vi "FractalNet BaseStation with GPS Weather and Gesture Display.vi"() -> ()   [LabVIEW 2009]
doc: "This example demonstrates some fundamental concepts for the 3D picture control. Concepts covered include:\n\n-Object creation\n-Texturing\n-Object movement\n-Object hierarchy"
uses:
  <vilib>/Utility/miscctls.llb/LVRectTypeDef.ctl
  <vilib>/Instr/_visa.llb/VISA Configure Serial Port (Instr).vi
  <vilib>/regexp/Match Regular Expression.xnode
  <vilib>/Analysis/coordinate.llb/3D Cartesian Coordinate Rotation (Euler) (Array).vi
  <vilib>/picture/3D Picture Control/NI_3D Picture Control.lvlib
  <vilib>/Analysis/NI_AALPro.lvlib
  <vilib>/Platform/NI_3dgraph.lvlib
panel:
  in  "3D Surface":refnum<k7>(container)
  out "Thermometer":dbl(slide) scale=0.0..100.0
  out "Status":dbl(knob)=5.599555604389847 scale=0.0..10.0
  in  "Boolean 7":bool
  out "Boolean 6":bool
  out "Boolean 5":bool
  out "Boolean 4":bool
  in  "Boolean 3":bool=TRUE
  in  "Boolean 2":bool=TRUE
  in  "Boolean":bool
  in  "Control":dbl(knob)=2.859770666370601 scale=0.0..10.0
  out "DENIO - CAVE 1":dbl(knob) scale=600.0..480.0
  out "GREENE - CAVE 2":dbl(knob) scale=600.0..480.0
  out "VAUGHN - SHIP":dbl(knob) scale=600.0..480.0
  in  "Acquire Glove":bool
  out "Date":string
  out "Base Heading (degrees)":dbl
  out "Base speed (mph)":dbl
  out "Time":string
  out "Longitude":string
  out "Latitude":string
  out "# of satellites":string
  out "Altitude (ft)":string
  out "Outside Pressure":string
  out "Outside Temp (F)":string
  out "Outside Temp (C)":string
  out "Outside Humidity":string
  in  "COMM for GPS / Weather":refnum<visa-resource-name>="COM22"
  in  "VISA Resource Name":refnum<visa-resource-name>="COM24"
  out "Raw DataGlove String":string
  out "Yaw":string
  out "Pitch":string
  out "Roll":string
  out "Heart":string
  out "Thumb":dbl(slide) scale=780.0..815.0
  out "Index":dbl(slide) scale=518.0..735.0
  out "Middle":dbl(slide) scale=780.0..880.0
  out "Ring":dbl(slide) scale=720.0..870.0
  in  "Render Dest":enum16{"Scene Window", "Scene Display"}(ring)=enum."Scene Display"
  in  "Camera Controller":enum16{"None", "Spherical", "Flying"}(ring)=enum."Spherical"
  out "Scene Display":refnum<vi>(3d-picture)
  out "error out":errorcluster
  in  "stop":bool
  # "NODE MAP STATUS"
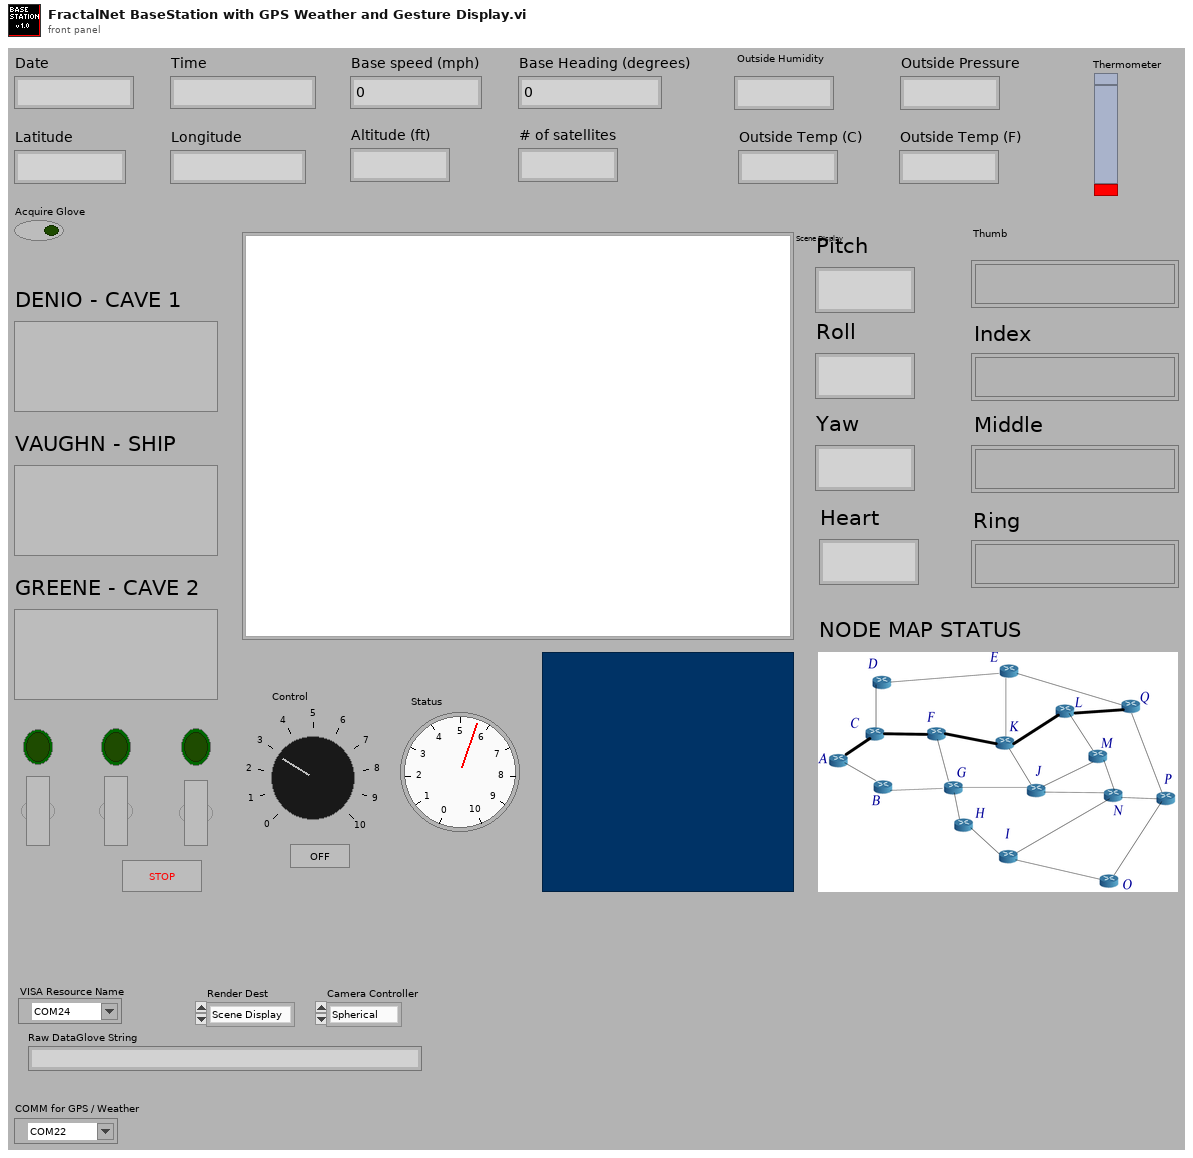
[diagram p1: front panel]
types:
  T1 = typedef "LVRectTypeDef.ctl" = cluster{"Left":i16, "Top":i16, "Right":i16, "Bottom":i16}
  T2 = enum16{"Open", "Minimized", "Maximized", "Hidden"}
  T3 = enum16{"As a Decal", "With Modulation", "With Blending", "As a replacement"}
  T4 = typedef "imagedata.ctl" = cluster{"image type":i32, "image depth":i32, "image":u8[], "mask":u8[], "colors":u32[], "Rectangle":cluster{"left":i16, "top":i16, "right":i16, "bottom":i16}}
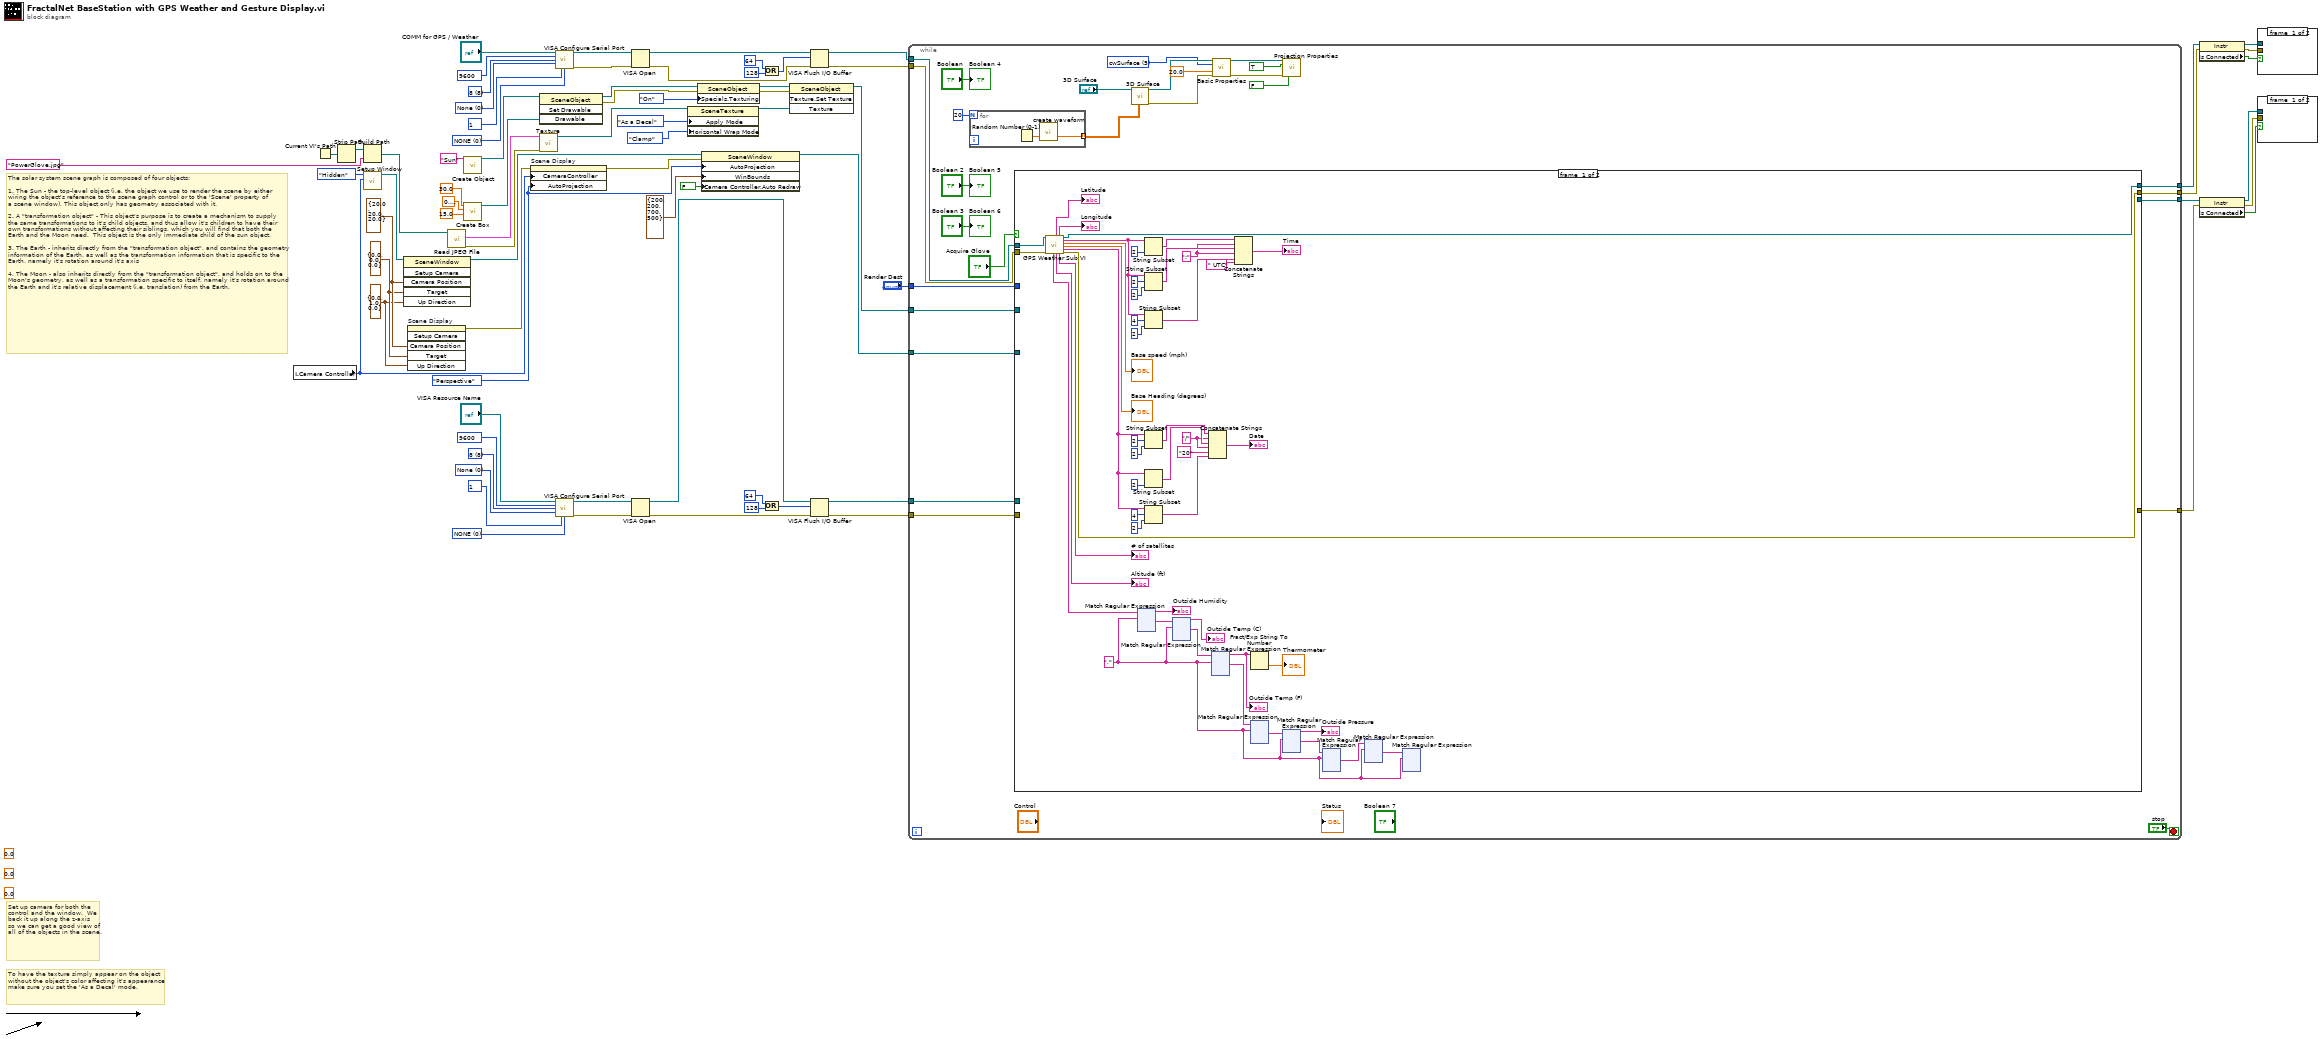
[diagram p0: block diagram]
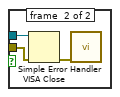
[diagram p2: hidden frame]
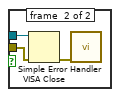
[diagram p3: hidden frame]
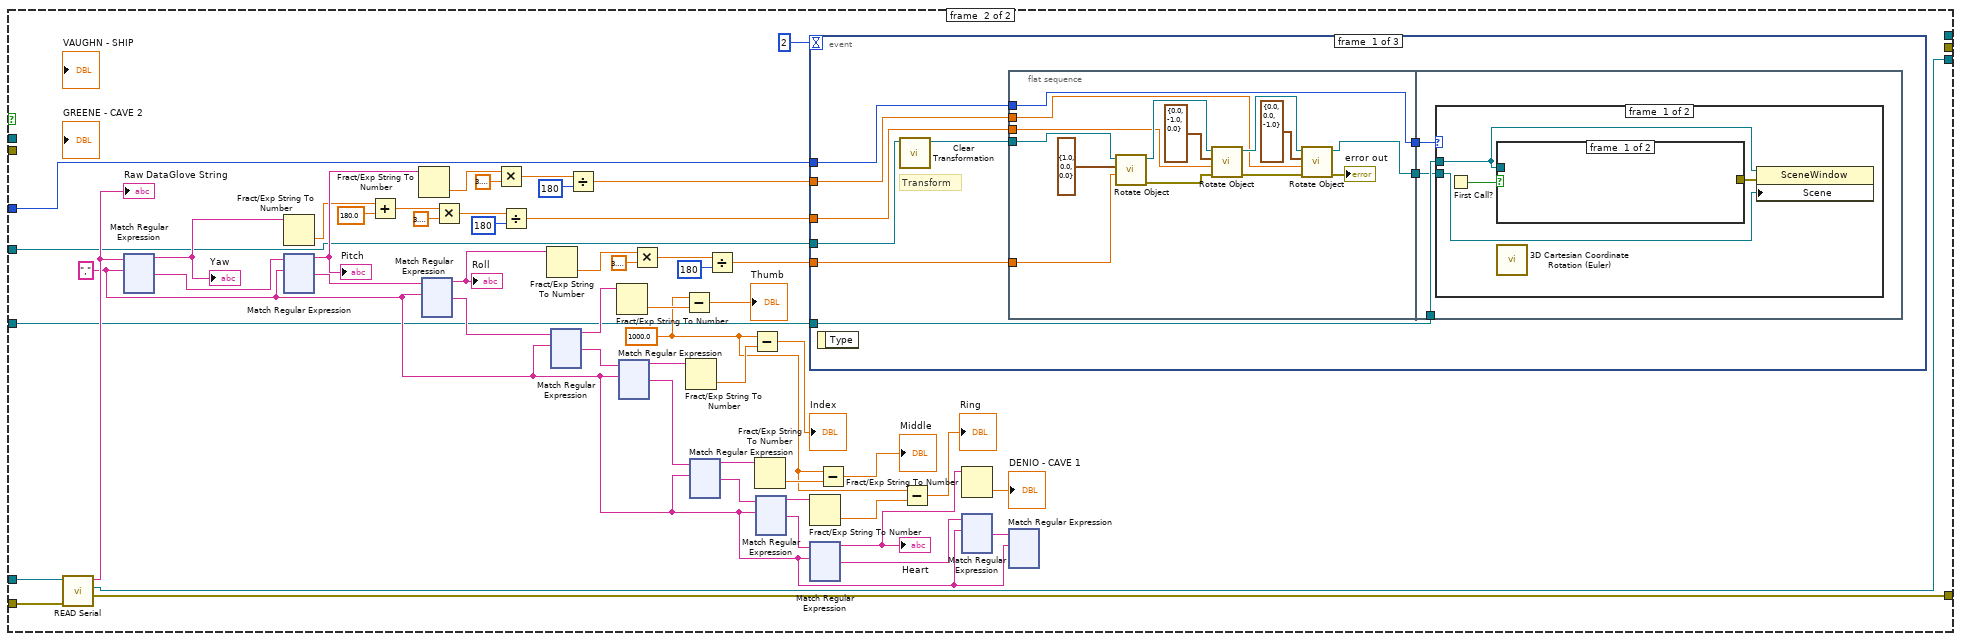
[diagram p4: hidden frame]
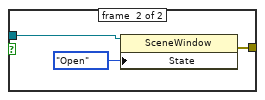
[diagram p5: hidden frame]
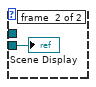
[diagram p6: hidden frame]
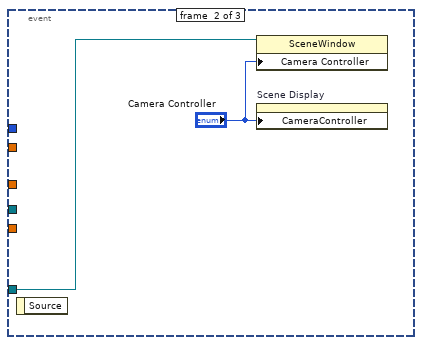
[diagram p7: hidden frame]
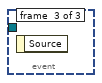
[diagram p8: hidden frame]
diagram:
  w13 = u16 0 items=["NONE", "XON/XOFF", "RTS/CTS", "XON/XOFF & RTS/CTS", "DTR/DSR", "XON/XOFF & DTR/DSR"] ("flow control")
  w14 = u16 10 items=["1"=10, "1.5"=15, "2"=20] ("stop bits")
  w15 = u16 0 items=["None", "Odd", "Even", "Mark", "Space"] ("parity")
  w16 = u16 8 items=["8"=8, "7"=7, "6"=6, "5"=5] ("data bits")
  w17 = u32 9600 items=["1200"=1200, "2400"=2400, "4800"=4800, "9600"=9600, "19200"=19200, "38400"=38400, "57600"=57600, "115200"=115200] ("baud rate")
  (unwired) 0.0
  (unwired) 0.0
  (unwired) 0.0
  w34 = u16 0 items=["NONE", "XON/XOFF", "RTS/CTS", "XON/XOFF & RTS/CTS", "DTR/DSR", "XON/XOFF & DTR/DSR"] ("flow control")
  w35 = u16 10 items=["1"=10, "1.5"=15, "2"=20] ("stop bits")
  w36 = u16 0 items=["None", "Odd", "Even", "Mark", "Space"] ("parity")
  w37 = u16 8 items=["8"=8, "7"=7, "6"=6, "5"=5] ("data bits")
  w38 = u32 9600 items=["1200"=1200, "2400"=2400, "4800"=4800, "9600"=9600, "19200"=19200, "38400"=38400, "57600"=57600, "115200"=115200] ("baud rate")
  w53 = enum16{"None", "Perspective", "Orthographic"}."Perspective" ("Auto Projection Mode")
  w56 = cluster{"X":sgl, "Y":sgl, "Z":sgl} {"X"=0.0, "Y"=1.0, "Z"=0.0} ("Up Direction")
  w57 = cluster{"X":sgl, "Y":sgl, "Z":sgl} {"X"=0.0, "Y"=0.0, "Z"=0.0} ("Target")
  w58 = cluster{"X":sgl, "Y":sgl, "Z":sgl} {"X"=20.0, "Y"=20.0, "Z"=20.0} ("Camera Position")
  # "Set up camera for both the \ncontrol and the window.  We\nback it up along the z-axis\nso we can get a good view of\nall of the objects in the scene."
  # "To have the texture simply appear on the object\nwithout the object's color affecting it's appearance\nmake sure you set the 'As a Decal' mode."
  # "The solar system scene graph is composed of four objects:\n\n1. The Sun - the top-level object (i.e. the object we use to render the scene by either\nwiring the object's reference to the scene graph control or to the 'Scene' property of \na scene window). This object only has geometry associated with it.\n\n2. A \"transformation object\" - This object's purpose is to create a mechanism to supply\nthe same transformations to it's child objects, and thus allow it's children to have their\nown transformations without affecting their siblings, which you will find that both the \nEarth and the Moon need.  This object is the only immediate child of the sun object.\n\n3. The Earth - inherits directly from the \"transformation object\", and contains the geometry\ninformation of the Earth, as well as the transformation information that is specific to the \nEarth, namely it's rotation around it's axis\n\n4. The Moon - also inherits directly from the \"transformation object\", and holds on to the \nMoon's geometry, as well as a transformation specific to itself, namely it's rotation around\nthe Earth and it's relative displacement (i.e. translation) from the Earth."
  n1 = local read "Camera Controller"() -> (w49:enum16{"None", "Spherical", "Flying"})
  n2 = Current VI's Path() -> (path=w63:path)
  n3 = Strip Path(path=w63) -> (stripped path=w62:path)  [unwired: 1 out]
  n4 = Build Path(base path=w62, name or relative path="PowerGlove.jpg" ("Name")) -> (appended path=w60:path)
  n5 = call <vilib>:"Setup Window.vi"("Camera Controller"=w49, "Window State"=T2."Hidden") -> ("New Window Refnum"=w51:refnum<vi>)  [unwired: 1 in, 8 out]
  n6 = invoke class="SceneWindow" method="Setup Camera"(reference=w51, "Camera Position"=w58, "Target"=w57, "Up Direction"=w56) -> (reference out=w76:refnum<vi>)  [unwired: 2 in, 5 out]
  n7 = invoke on="Scene Display" class="SceneGraphDisp (strict)" method="Setup Camera"("Camera Position"=w58, "Target"=w57, "Up Direction"=w56) -> (error out=w55:errorcluster)  [unwired: 3 in, 5 out]
  n8 = call <vilib>:"Read JPEG File.vi"("path to JPEG file"=w60) -> ("error out"=w72:errorcluster, "image data"=w73:T4)  [unwired: 1 in, 8 out]
  n9 = call <vilib>:"Create Object.vi"("Name"="Sun") -> ("Scene:New Object"=w74:refnum<vi>)  [unwired: 1 in, 9 out]
  n10 = call <vilib>:"Create Box.vi"("Length Z"=sgl 15.0, "Length Y"=sgl 0.1, "Length X"=sgl 30.0) -> ("New Box Refnum"=w42:refnum<vi>)  [unwired: 7 in, 1 out]
  n11 = property on="Scene Display" class="SceneGraphDisp (strict)"(error in=w55, "CameraController"=w49, "AutoProjection"=w53) -> (error out=w54:errorcluster)  [unwired: 1 in, 1 out]
  n12 = call <vilib>:"Texture.vi"("error in (no error)"=w72, "Image"=w73) -> ("New Texture Refnum"=w66:refnum<vi>)  [unwired: 9 out]
  n13 = invoke class="SceneObject" method="Set Drawable"(reference=w74, "Drawable"=w42) -> (reference out=w71:refnum<vi>, error out=w69:errorcluster)  [unwired: 2 in, 2 out]
  n14 = call-poly "VISA Configure Serial Port"("VISA resource name"="COMM for GPS / Weather", "baud rate (9600)"=w17, "data bits (8)"=w16, "parity (0:none)"=w15, "stop bits (10: 1 bit)"=w14, "flow control (0:none)"=w13) -> ("VISA resource name out"=w20:refnum<visa-resource-name>, "error out"=w19:errorcluster)  [unwired: 1 in, 7 out]
  n15 = call-poly "VISA Configure Serial Port"("VISA resource name"="VISA Resource Name", "baud rate (9600)"=w38, "data bits (8)"=w37, "parity (0:none)"=w36, "stop bits (10: 1 bit)"=w35, "flow control (0:none)"=w34) -> ("VISA resource name out"=w41:refnum<visa-resource-name>, "error out"=w40:errorcluster)  [unwired: 1 in, 7 out]
  n16 = VISA Open(error in (no error)=w19, VISA resource name=w20) -> (VISA resource name=w12:refnum<visa-resource-name>, error out=w11:errorcluster)  [unwired: 3 out]
  n17 = VISA Open(error in (no error)=w40, VISA resource name=w41) -> (VISA resource name=w33:refnum<visa-resource-name>, error out=w32:errorcluster)  [unwired: 3 out]
  n18 = property class="SceneTexture"(reference=w66, "Apply Mode"=T3."As a Decal", "Horizontal Wrap Mode"=enum16{"Clamp", "Repeat"}."Clamp") -> (reference out=w64:refnum<vi>)  [unwired: 1 in, 1 out]
  n19 = property class="SceneObject"(reference=w71, error in=w69, "Specials.Texturing"=enum16{"Inherit Value", "Off", "On"}."On" ("Specials:Texturing")) -> (reference out=w70:refnum<vi>, error out=w68:errorcluster)
  n20 = property class="SceneWindow"(reference=w76, error in=w54, "AutoProjection"=w53, "WinBounds"=T1 {"Left"=200, "Top"=200, "Right"=700, "Bottom"=500} ("Window Bounds"), "Camera Controller.Auto Redraw"=FALSE ("Camera Controller:Auto Redraw")) -> (reference out=w47:refnum<vi>)  [unwired: 1 out]
  n21 = Compound Arithmetic op=OR(64, 128) -> (w8:i32)
  n22 = Compound Arithmetic op=OR(64, 128) -> (w29:i32)
  n23 = invoke class="SceneObject" method="Texture.Set Texture"(reference=w70, error in=w68, "Texture"=w64) -> (reference out=w21:refnum<vi>)  [unwired: 1 in, 3 out]
  n24 = VISA Flush I/O Buffer(VISA resource name=w12, mask (16)=w8, error in (no error)=w11) -> (VISA resource name out=w7:refnum<visa-resource-name>, error out=w6:errorcluster)
  n25 = VISA Flush I/O Buffer(VISA resource name=w33, mask (16)=w29, error in (no error)=w32) -> (VISA resource name out=w23:refnum<visa-resource-name>, error out=w22:errorcluster)
  n26 = while {
    tunnel: w47 -> [w97]
    tunnel: "Render Dest" -> [w103]
    tunnel: w21 -> [w98]
    tunnel: [w102] -> w25
    tunnel: [w101] -> w24
    tunnel: w23 -> [w100]
    tunnel: w22 -> [w99]
    tunnel: w7 -> [w95]
    tunnel: w6 -> [w94]
    tunnel: [w93] -> w2
    tunnel: [w92] -> w1
    stop <- "stop" stop-if-true
    w80 = 5 items=["cwLine"=1, "cwPoint"=2, "cwLinePoint"=3, "cwHiddenLine"=4, "cwSurface"=5, "cwSurfaceLine"=6, "cwSurfaceNormal"=7, "cwContourLine"=8, "cwSurfaceContour"=9] ("Plot Style")
    n27 = for {
      N: 20 -> [_]
      tunnel: [w104] -> w84 mode=indexing
      n28 = Random Number (0-1)() -> (number: 0 to 1=w105:dbl)
      n29 = call "create waveform.vi"("amplitude (1.0)"=w105) -> ("waveform graph"=w104:ext[])  [unwired: 13 in, 1 out]
    }
    n30 = case shown="False" "Acquire Glove" {
      tunnel: w103 -> [_ w1062]
      tunnel: [_ w1061] -> w102
      tunnel: [_ w1060] -> w101
      tunnel: w100 -> [_ w1059]
      tunnel: w99 -> [_ w1058]
      tunnel: w98 -> [_ w1013]
      tunnel: w97 -> [_ w1012]
      tunnel: w95 -> [w112 _]
      tunnel: w94 -> [w111 _]
      tunnel: [w110 _] -> w93
      tunnel: [w109 _] -> w92
      frame #0 {
        w147 = "/" ("string")
        w133 = ":" ("string")
        w138 = "," ("regular expression")
        n31 = call "GPS Weather Sub VI.vi"("VISA resource name out"=w112, "error out"=w111) -> ("Weather"=w141:string, "Latitude"=→"Latitude":string, "Altitude"=→"Altitude (ft)":string, "Longitude"=→"Longitude":string, "# of satellites"=→"# of satellites":string, "VISA resource name out 2"=w110:refnum<visa-resource-name>, "Time"=w130:string, "Base speed (mph)"=→"Base speed (mph)":dbl, "Base Heading (degrees)"=→"Base Heading (degrees)":dbl, "Date"=w148:string, "error IO"=w109:errorcluster)  [unwired: 7 in]
        n32 = xnode "Match Regular Expression"("input string"=w141, "regular expression"=w138) -> ("before match"=→"Outside Humidity":string, "after match"=w119:string)  [unwired: 2 in, 5 out]
        n33 = String Subset(string=w130, length (rest)=2 ("length (rest)")) -> (substring=w132:string)  [unwired: 1 in]
        n34 = String Subset(string=w130, offset (0)=2, length (rest)=2 ("length (rest)")) -> (substring=w134:string)
        n35 = String Subset(string=w130, offset (0)=4, length (rest)=2 ("length (rest)")) -> (substring=w135:string)
        n36 = String Subset(string=w148, offset (0)=2, length (rest)=2 ("length (rest)")) -> (substring=w149:string)
        n37 = String Subset(string=w148, length (rest)=2 ("length (rest)")) -> (substring=w150:string)  [unwired: 1 in]
        n38 = String Subset(string=w148, offset (0)=4, length (rest)=2 ("length (rest)")) -> (substring=w152:string)
        n39 = xnode "Match Regular Expression"("input string"=w119, "regular expression"=w138) -> ("before match"=→"Outside Temp (C)":string, "after match"=w118:string)  [unwired: 2 in, 5 out]
        n40 = Concatenate Strings(w149, w147, w150, w147, "20" ("string"), w152) -> (→"Date":string)
        n41 = xnode "Match Regular Expression"("input string"=w118, "regular expression"=w138) -> ("before match"=w106:string, "after match"=w117:string)  [unwired: 2 in, 5 out]
        "Outside Temp (F)" <- w106
        n42 = Concatenate Strings(w132, w133, w134, w133, w135, " UTC" ("string")) -> (→"Time":string)
        n43 = Fract/Exp String To Number(string=w106) -> (number=→"Thermometer":dbl)  [unwired: 3 in, 1 out]
        n44 = xnode "Match Regular Expression"("input string"=w117, "regular expression"=w138) -> ("after match"=w116:string)  [unwired: 2 in, 6 out]
        n45 = xnode "Match Regular Expression"("input string"=w116, "regular expression"=w138) -> ("before match"=→"Outside Pressure":string, "after match"=w115:string)  [unwired: 2 in, 5 out]
        n46 = xnode "Match Regular Expression"("input string"=w115, "regular expression"=w138) -> ("after match"=w114:string)  [unwired: 2 in, 6 out]
        n47 = xnode "Match Regular Expression"("input string"=w114, "regular expression"=w138) -> ("after match"=w113:string)  [unwired: 2 in, 6 out]
        n48 = xnode "Match Regular Expression"("input string"=w113, "regular expression"=w138) -> ()  [unwired: 2 in, 7 out]
      }
      frame #1 {
        w1036 = 1000.0 ("x")
        w1034 = "," ("regular expression")
        n49 = call "READ Serial.vi"("error in"=w1058, "VISA Resource Name In"=w1059) -> ("error out"=w1060:errorcluster, "VISA Resource Name Out"=w1061:refnum<visa-resource-name>, "Output String"=w1048:string)  [unwired: 4 in]
        "Raw DataGlove String" <- w1048
        n50 = xnode "Match Regular Expression"("input string"=w1048, "regular expression"=w1034) -> ("before match"=w1020:string, "after match"=w1057:string)  [unwired: 2 in, 5 out]
        "Yaw" <- w1020
        n51 = Fract/Exp String To Number(string=w1020) -> (number=w1016:dbl)  [unwired: 3 in, 1 out]
        n52 = xnode "Match Regular Expression"("input string"=w1057, "regular expression"=w1034) -> ("before match"=w1033:string, "after match"=w1056:string)  [unwired: 2 in, 5 out]
        "Pitch" <- w1033
        n53 = Add(x=w1016, y=180.0) -> (x+y=w1014:dbl)
        n54 = Fract/Exp String To Number(string=w1033) -> (number=w1022:dbl)  [unwired: 3 in, 1 out]
        n55 = xnode "Match Regular Expression"("input string"=w1056, "regular expression"=w1034) -> ("before match"=w1032:string, "after match"=w1055:string)  [unwired: 2 in, 5 out]
        "Roll" <- w1032
        n56 = Multiply(x=w1014, y=3.141592653589793) -> (x*y=w1030:dbl)
        n57 = Multiply(x=w1022, y=3.141592653589793) -> (x*y=w1027:dbl)
        n58 = Divide(x=w1030, y=180) -> (x/y=w1017:dbl)
        n59 = Fract/Exp String To Number(string=w1032) -> (number=w1021:dbl)  [unwired: 3 in, 1 out]
        n60 = xnode "Match Regular Expression"("input string"=w1055, "regular expression"=w1034) -> ("before match"=w1047:string, "after match"=w1050:string)  [unwired: 2 in, 5 out]
        n61 = Divide(x=w1027, y=180) -> (x/y=w1019:dbl)
        n62 = Fract/Exp String To Number(string=w1047) -> (number=w1046:dbl)  [unwired: 3 in, 1 out]
        n63 = xnode "Match Regular Expression"("input string"=w1050, "regular expression"=w1034) -> ("before match"=w1044:string, "after match"=w1054:string)  [unwired: 2 in, 5 out]
        n64 = Multiply(x=w1021, y=3.141592653589793) -> (x*y=w1024:dbl)
        n65 = Subtract(x=w1036, y=w1046) -> (x-y=→"Thumb":dbl)
        n66 = Fract/Exp String To Number(string=w1044) -> (number=w1043:dbl)  [unwired: 3 in, 1 out]
        n67 = xnode "Match Regular Expression"("input string"=w1054, "regular expression"=w1034) -> ("before match"=w1037:string, "after match"=w1053:string)  [unwired: 2 in, 5 out]
        n68 = Divide(x=w1024, y=180) -> (x/y=w1018:dbl)
        n69 = Subtract(x=w1036, y=w1043) -> (x-y=→"Index":dbl)
        n70 = Fract/Exp String To Number(string=w1037) -> (number=w1039:dbl)  [unwired: 3 in, 1 out]
        n71 = xnode "Match Regular Expression"("input string"=w1053, "regular expression"=w1034) -> ("before match"=w1040:string, "after match"=w1052:string)  [unwired: 2 in, 5 out]
        n72 = event shown="[2] \"stop\": Value Change" {
          selector: _ -> [_ _ _]
          dyn-events: _ -> [_ _ _]
          timeout: 2 -> [_ _ _]
          tunnel: w1012 -> [w2142 w2169 _]
          tunnel: w1062 -> [w2140 _ _]
          tunnel: w1013 -> [w2135 _ _]
          tunnel: w1017 -> [w2138 _ _]
          tunnel: w1018 -> [w2137 _ _]
          tunnel: w1019 -> [w2136 _ _]
          event #0 {
            # "Transform"
            n73 = event-data() -> ()  [unwired: 2 out]
            n74 = call <vilib>:"Clear Transformation.vi"("Object Refnum In"=w2135) -> ("Object Refnum Out"=w2134:refnum<vi>)  [unwired: 9 in, 1 out]
            n75 = flat-sequence {
              tunnel: w2134 -> [w2149]
              tunnel: [w2156] -> w2141
              tunnel: w2140 -> [w2156]
              tunnel: [w2150] -> w2139
              tunnel: w2138 -> [w2144]
              tunnel: w2137 -> [w2145]
              tunnel: w2136 -> [w2143]
              tunnel: w2142 -> [w2159]
              tunnel: w2141 -> [w2158]
              tunnel: w2139 -> [w2157]
              frame #0 {
                n76 = call <vilib>:"Rotate Object.vi"("Angle"=w2145, "Axis"=cluster{"X":sgl, "Y":sgl, "Z":sgl} {"X"=1.0, "Y"=0.0, "Z"=0.0}, "Scene.Object In"=w2149) -> ("error out"=w2147:errorcluster, "Scene.Object Out"=w2146:refnum<vi>)  [unwired: 7 in]
                n77 = call <vilib>:"Rotate Object.vi"("error in (no error)"=w2147, "Angle"=w2144, "Axis"=cluster{"X":sgl, "Y":sgl, "Z":sgl} {"X"=0.0, "Y"=-1.0, "Z"=0.0}, "Scene.Object In"=w2146) -> ("error out"=w2152:errorcluster, "Scene.Object Out"=w2153:refnum<vi>)  [unwired: 6 in]
                n78 = call <vilib>:"Rotate Object.vi"("error in (no error)"=w2152, "Angle"=w2143, "Axis"=cluster{"X":sgl, "Y":sgl, "Z":sgl} {"X"=0.0, "Y"=0.0, "Z"=-1.0}, "Scene.Object In"=w2153) -> ("error out"=→"error out":errorcluster, "Scene.Object Out"=w2150:refnum<vi>)  [unwired: 6 in]
              }
              frame #1 {
                n79 = case shown="\"Scene Window\", Default" w2158 {
                  tunnel: w2159 -> [w2163 _]
                  tunnel: w2157 -> [w2160 w2167]
                  frame #0 {
                    n80 = First Call?() -> (First Call?: T/F=w2161:bool)
                    n81 = case shown="True" w2161 {
                      tunnel: w2163 -> [_ w2166]
                      tunnel: [_ w2165] -> w2162
                      frame #0 {
                      }
                      frame #1 {
                        n82 = property class="SceneWindow"(reference=w2166, "State"=T2."Open" ("Window State")) -> (error out=w2165:errorcluster)  [unwired: 1 in, 1 out]
                      }
                    }
                    n83 = call-poly <vilib>:"3D Cartesian Coordinate Rotation (Euler).vi"() -> ()  [unwired: 8 in, 4 out]
                    n84 = property class="SceneWindow"(reference=w2163, error in=w2162, "Scene"=w2160) -> ()  [unwired: 2 out]
                  }
                  frame #1 {
                    "Scene Display" <- w2167
                  }
                }
              }
            }
          }
          event #1 {
            n85 = event-data() -> ()  [unwired: 2 out]
            n86 = property class="SceneWindow"(reference=w2169, "Camera Controller"="Camera Controller") -> ()  [unwired: 1 in, 2 out]
            n87 = property on="Scene Display" class="SceneGraphDisp (strict)"("CameraController"="Camera Controller") -> ()  [unwired: 2 in, 2 out]
          }
          event #2 {
            n88 = event-data() -> ()  [unwired: 2 out]
          }
        }
        n89 = Fract/Exp String To Number(string=w1040) -> (number=w1041:dbl)  [unwired: 3 in, 1 out]
        n90 = xnode "Match Regular Expression"("input string"=w1052, "regular expression"=w1034) -> ("before match"=w1011:string, "after match"=w1051:string)  [unwired: 2 in, 5 out]
        "Heart" <- w1011
        n91 = Subtract(x=w1036, y=w1039) -> (x-y=→"Middle":dbl)
        n92 = Subtract(x=w1036, y=w1041) -> (x-y=→"Ring":dbl)
        n93 = Fract/Exp String To Number(string=w1011) -> (number=→"DENIO - CAVE 1":dbl)  [unwired: 3 in, 1 out]
        n94 = xnode "Match Regular Expression"("input string"=w1051, "regular expression"=w1034) -> ("after match"=w1049:string)  [unwired: 2 in, 6 out]
        n95 = xnode "Match Regular Expression"("input string"=w1049, "regular expression"=w1034) -> ()  [unwired: 2 in, 7 out]
      }
    }
    n96 = call <vilib>:"3D Surface.vi"("z matrix"=w84, "3D graph"="3D Surface") -> ("error out"=w86:errorcluster, "3D graph out"=w87:refnum<k7>)  [unwired: 8 in]
    n97 = call <vilib>:"Basic Properties.vi"("3D graph"=w87, "plot style"=w80, "transparency"=20.0 ("Transparency (%)"), "error in (no error)"=w86) -> ("3D graph out"=w83:refnum<k7>, "error out"=w82:errorcluster)  [unwired: 10 in]
    n98 = call <vilib>:"Projection Properties.vi"("3D graph"=w83, "xy projection"=TRUE ("XY Projection"), "error in (no error)"=w82, "show projections only"=FALSE ("Show Projections Only")) -> ()  [unwired: 10 in, 2 out]
    "Boolean 4" <- "Boolean"
    "Boolean 5" <- "Boolean 2"
    "Boolean 6" <- "Boolean 3"
  }
  n99 = property class="Instr"(reference=w2, error in=w1) -> (reference out=w3:refnum<visa-resource-name>, error out=w4:errorcluster, "Is Connected"=w5:bool)
  n100 = property class="Instr"(reference=w25, error in=w24) -> (reference out=w28:refnum<visa-resource-name>, error out=w27:errorcluster, "Is Connected"=w26:bool)
  n101 = case shown="True" w5 {
    tunnel: w3 -> [_ w2172]
    tunnel: w4 -> [_ w2171]
    frame #0 {
    }
    frame #1 {
      n102 = VISA Close(VISA resource name=w2172, error in (no error)=w2171) -> (error out=w2170:errorcluster)
      n103 = call <vilib>:"Simple Error Handler.vi"("error in (no error)"=w2170) -> ()  [unwired: 1 in, 8 out]
    }
  }
  n104 = case shown="True" w26 {
    tunnel: w28 -> [_ w2175]
    tunnel: w27 -> [_ w2174]
    frame #0 {
    }
    frame #1 {
      n105 = VISA Close(VISA resource name=w2175, error in (no error)=w2174) -> (error out=w2173:errorcluster)
      n106 = call <vilib>:"Simple Error Handler.vi"("error in (no error)"=w2173) -> ()  [unwired: 1 in, 8 out]
    }
  }
